vi "Group by Parent.vi"(11 "List of Runnables":string[](array[string])) -> (3 "Methods":cluster{"Methods":string[]}[](array[cluster]))   [LabVIEW 2020, in "Parallell Test Runner.lvclass"]
uses:
  Parallell Test Runner.lvclass
  <vilib>/Utility/miscctls.llb/LVMapReplaceAction.ctl
panel:
  out "map":map{string, string[]}(c390)
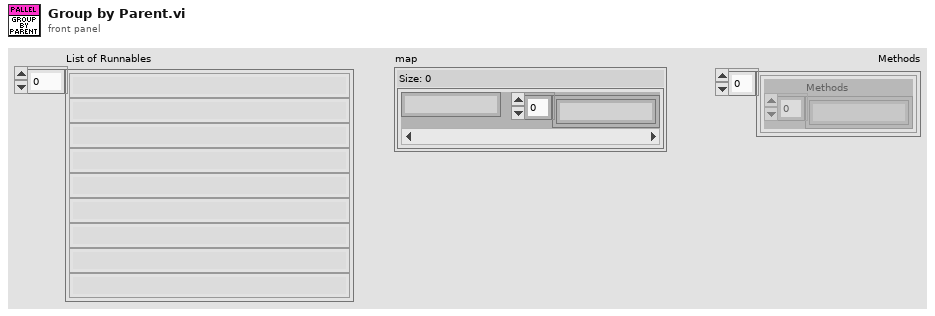
[diagram p1: front panel]
types:
  T1 = typedef "LVMapReplaceAction.ctl" = enum32{"Modify Entry only if found", "Add or Modify Entry", "Delete Entry"}
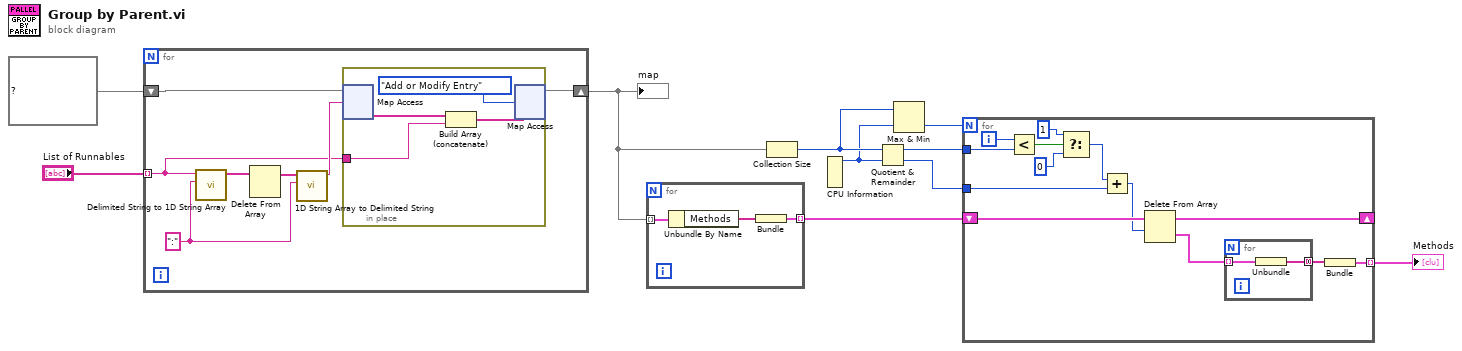
[diagram p0: block diagram]
diagram:
  n1 = for {
    tunnel: "List of Runnables" -> [w12] mode=indexing
    shift-right: [w11] -> w8
    shift-left: map{string, string[]} {} ("map") -> [w17]
    w14 = ":" ("delimiter")
    n2 = call <vilib>:"Delimited String to 1D String Array.vi"("delimiter"=w14, "delimited string"=w12) -> ("string array"=w16:string[])  [unwired: 9 in]
    n3 = Delete From Array(array=w16) -> (array with subset deleted=w15:string[])  [unwired: 2 in, 1 out]
    n4 = call <vilib>:"1D String Array to Delimited String.vi"("delimiter"=w14, "string array"=w15) -> ("delimited string"=w13:string)  [unwired: 9 in]
    n5 = in-place {
      in-place-border: w12 -> [w19]
      n6 = in-place-map #1(w17, w13) -> (w21:string[])  [unwired: 1 in, 1 out]
      n7 = Build Array (concatenate)(w21, w19) -> (w20:string[])
      n8 = in-place-map #1(w20, LVMapReplaceAction."Add or Modify Entry" ("action")) -> (w11:map{string, string[]})  [unwired: 2 out]
    }
  }
  "map" <- w8
  n9 = for {
    tunnel: w8 -> [w24] mode=indexing
    tunnel: [w22] -> w4 mode=indexing
    n10 = Unbundle By Name(w24) -> ("Methods"=w23:string[])
    n11 = Bundle("Methods"=w23) -> (w22:cluster{"Methods":string[]})  [unwired: 1 in]
  }
  n12 = Collection Size(1:w8) -> (0:w3:i32)
  n13 = CPU Information() -> (4:w2:i32)  [unwired: 3 out]
  n14 = Quotient & Remainder(x=w3, y=w2) -> (x-y*floor(x/y)=w7:i32, floor(x/y)=w6:i32)
  n15 = Max & Min(x=w3, y=w2) -> (min(x,y)=w1:i32)  [unwired: 1 out]
  n16 = for {
    N: w1 -> [_]
    tunnel: [w32] -> w5 mode=indexing
    tunnel: w7 -> [w36]
    tunnel: w6 -> [w34]
    shift-right: [w25] -> _
    shift-left: w4 -> [w37]
    i -> [w35]
    n17 = Less?(x=w35, y=w36) -> (x < y?=w31:bool)
    n18 = Select(t=1 ("x*y"), s=w31, f=0 ("x*y")) -> (s? t:f=w30:i32)
    n19 = Add(x=w30, y=w34) -> (x+y=w27:i32)
    n20 = Delete From Array(array=w37, length=w27) -> (deleted portion=w26:cluster{"Methods":string[]}[], array with subset deleted=w25:cluster{"Methods":string[]}[])  [unwired: 1 in]
    n21 = for {
      tunnel: w26 -> [w39] mode=indexing
      tunnel: [w38] -> w33 mode=concatenating
      n22 = Unbundle(w39) -> ("Methods"=w38:string[])
    }
    n23 = Bundle("Methods"=w33) -> (w32:cluster{"Methods":string[]})  [unwired: 1 in]
  }
  "Methods" <- w5
